vi "Configure Fixed Frequency.vi"(7 "Channel (1)":i32=1, 8 "error in (no error)":errorcluster, 10 "Fixed Frequency (300.0E+3)":dbl=300000.0 format="%^.2e", 11 "VISA resource name":refnum<visa-resource-name>) -> (0 "error out":errorcluster, 3 "VISA resource name out":refnum<visa-resource-name>)   [LabVIEW 2011, in "Agilent ENA Series.lvlib"]
doc: "This VI sets the fixed frequency (CW frequency) for the power sweep."
uses:
  Agilent ENA Series.lvlib
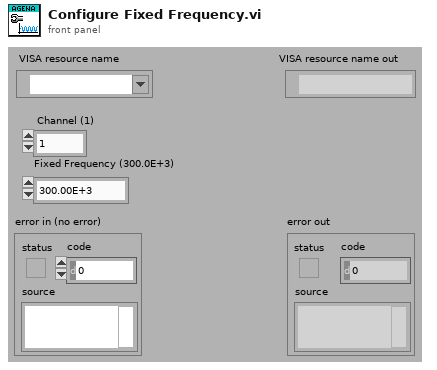
[diagram p1: front panel]
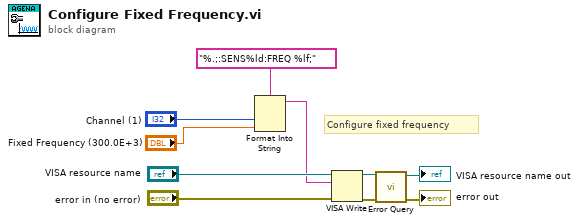
[diagram p0: block diagram]
diagram:
  # "Configure fixed frequency"
  n1 = Format Into String(format string="%.;:SENS%ld:FREQ %lf;", "Channel (1)", "Fixed Frequency (300.0E+3)") -> (resulting string=w5:string)  [unwired: 2 in, 1 out]
  n2 = VISA Write(VISA resource name="VISA resource name", write buffer=w5, error in (no error)="error in (no error)") -> (VISA resource name out=w4:refnum<visa-resource-name>, error out=w1:errorcluster)  [unwired: 1 out]
  n3 = call "Error Query.vi"("error in (no error)"=w1, "VISA resource name"=w4) -> ("error out"=→"error out":errorcluster, "VISA resource name out"=→"VISA resource name out":refnum<visa-resource-name>)  [unwired: 6 in, 2 out]
